vi "tearDown.vi"(8 "error in (no error)":errorcluster, 11 "fpMgr in":refnum<class "VIProviderShellHelper.lvclass">) -> (0 "error out":errorcluster, 3 "VI":refnum<vi>)   [LabVIEW 2019, in "LabVIEW-VIProviderShell.lvlib" / "VIProviderShellHelper.lvclass"]
uses:
  VIProviderShellHelper.lvclass
  VIProviderShellHelper.lvclass/VIProviderShellHelper.ctl
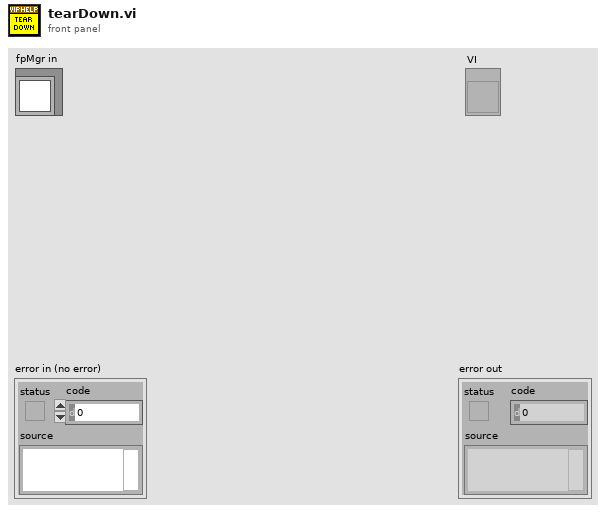
[diagram p1: front panel]
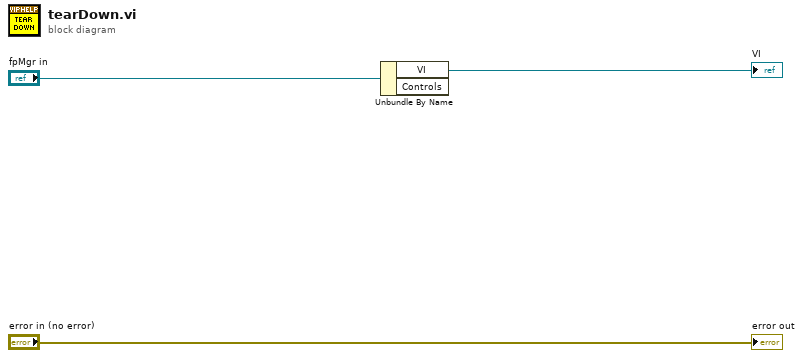
[diagram p0: block diagram]
diagram:
  n1 = Unbundle By Name("fpMgr in") -> ("VI"=→"VI":refnum<vi>)  [unwired: 1 out]
  "error out" <- "error in (no error)"
